vi "数据查询_仪器数据.vi"() -> ()   [LabVIEW 2016]
uses:
  <vilib>/Utility/miscctls.llb/LVRowAndColumnUnsignedTypeDef.ctl
  <vilib>/Utility/miscctls.llb/LVPointTypeDef.ctl
  SQL/database.lvlib
panel:
  in  "查询":bool
  in  "结束日期":string="2020/01/01"
  in  "起始日期":string="2010/01/01"
  in  "组合框":string(combo)
  out "数据表":string[][](table)
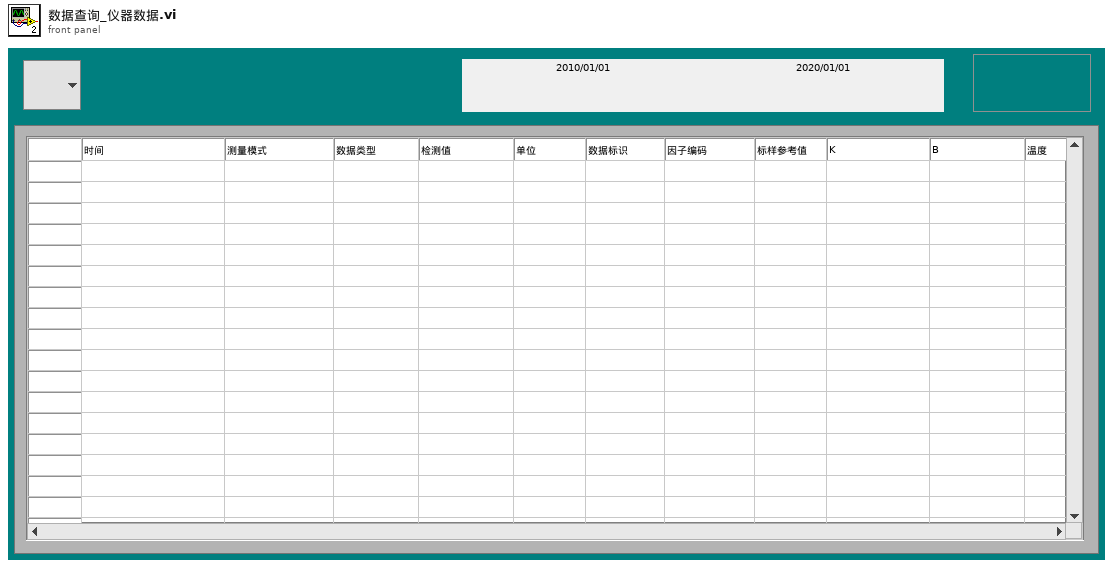
[diagram p1: front panel]
types:
  T1 = typedef "LVRowAndColumnUnsignedTypeDef.ctl" = cluster{"Row":u32, "Column":u32}
  T2 = typedef "LVPointTypeDef.ctl" = cluster{"Horizontal":i16, "Vertical":i16}
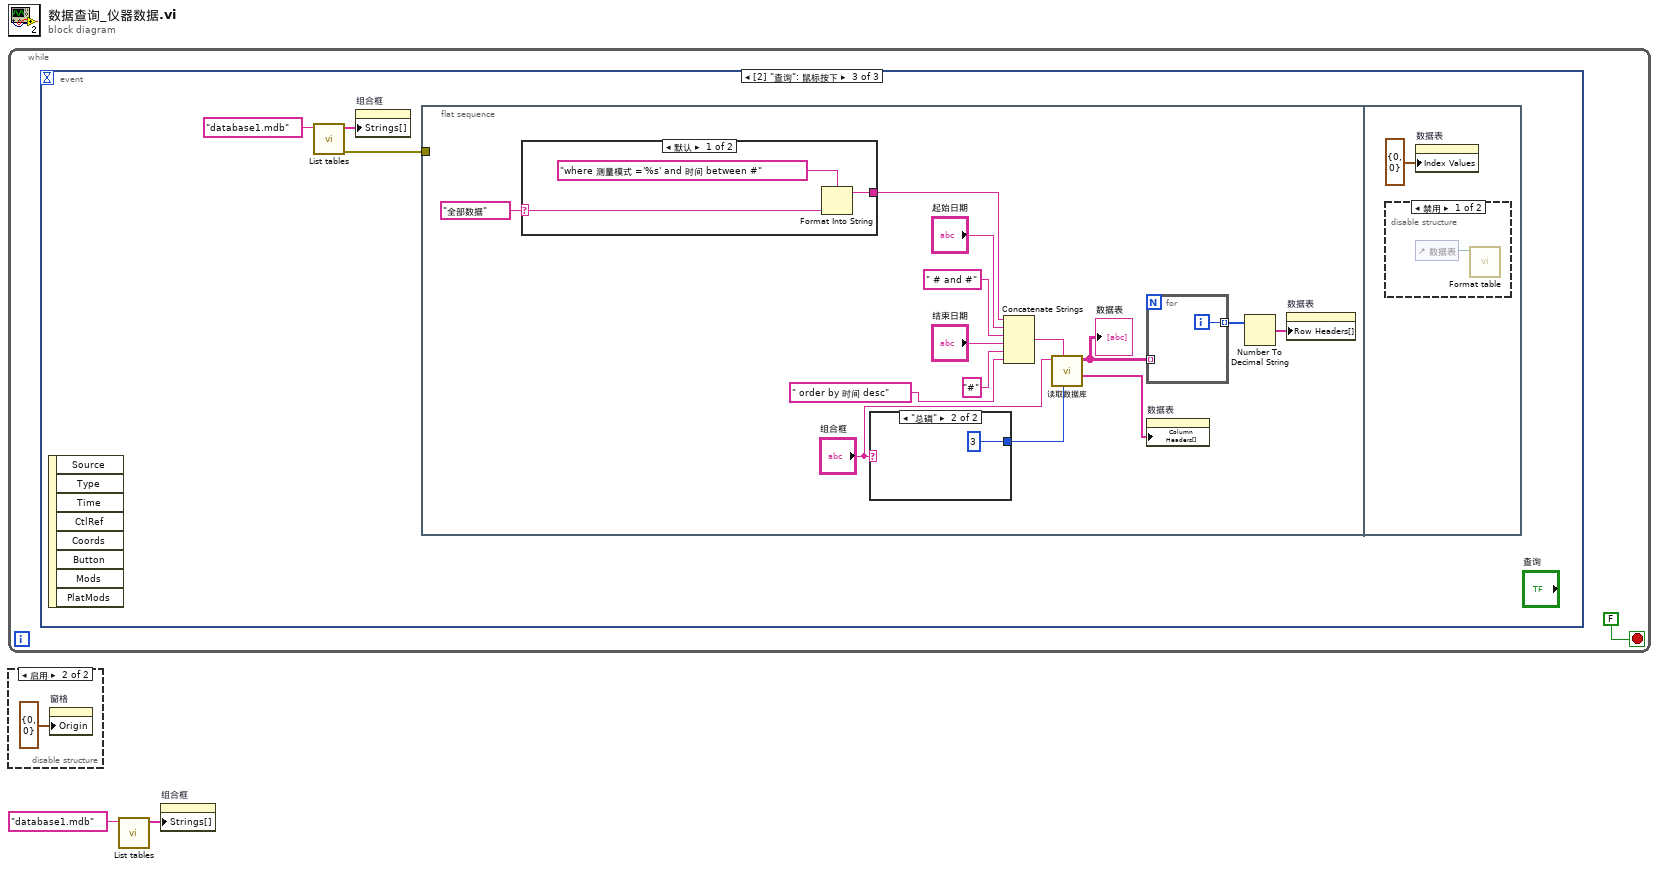
[diagram p0: block diagram]
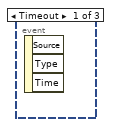
[diagram p2: hidden frame]
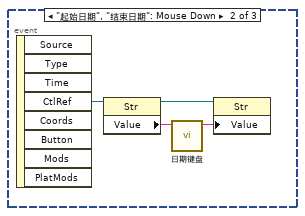
[diagram p3: hidden frame]
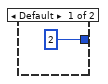
[diagram p4: hidden frame]
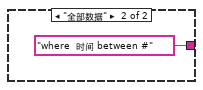
[diagram p5: hidden frame]
diagram:
  n1 = while {
    stop <- FALSE stop-if-true
    n2 = event shown="[2] \"查询\": 鼠标按下" {
      selector: _ -> [_ _ _]
      dyn-events: _ -> [_ _ _]
      timeout: _ -> [_ _ _]
      event Timeout {
        n3 = event-data() -> ()  [unwired: 1 in, 3 out]
      }
      event "起始日期", "结束日期": Mouse Down {
        n4 = event-data() -> ("CtlRef"=w7:refnum<vi>)  [unwired: 1 in, 7 out]
        n5 = property class="Str"(reference=w7) -> (reference out=w5:refnum<vi>, "Value"=w6:string)  [unwired: 1 in, 1 out]
        n6 = call "日期键盘.vi"("原值"=w6) -> ("x+y"=w4:string)  [unwired: 10 in]
        n7 = property class="Str"(reference=w5, "Value"=w4) -> ()  [unwired: 1 in, 2 out]
      }
      event "查询": Mouse Down {
        n8 = event-data() -> ()  [unwired: 1 in, 8 out]
        n9 = call "List tables.vi"("database"="database1.mdb") -> ("error out"=w8:errorcluster, "tables"=w10:string[])  [unwired: 9 in]
        n10 = property on="组合框" class="CmbBox"("Strings[]"=w10) -> ()  [unwired: 2 in, 2 out]
        n11 = flat-sequence {
          tunnel: w8 -> [_]
          frame #0 {
            n12 = case shown="默认" "全部数据" ("工作模式") {
              selector: "全部数据" ("工作模式") -> [w29 _]
              tunnel: [w27 "where  时间 between #" ("condition")] -> w13
              frame Default {
                n13 = Format Into String(format string="where 测量模式 ='%s' and 时间 between #" ("condition"), w29) -> (resulting string=w27:string)  [unwired: 2 in, 1 out]
              }
              frame "全部数据" {
              }
            }
            n14 = case shown="\"总磷\"" "组合框" {
              tunnel: [i16 2 ("精度(6)") i16 3 ("精度(6)")] -> w11
              frame Default {
              }
              frame "总磷" {
              }
            }
            n15 = Concatenate Strings(w13, "起始日期", " # and #" ("condition"), "结束日期", "#" ("condition"), " order by 时间 desc" ("字符串")) -> (w23:string)
            n16 = call "读取数据库.vi"("精度(6)"=w11, "condition"=w23, "组合框"="组合框") -> ("columns"=w19:string[], "表格"=w17:string[][])  [unwired: 5 in, 2 out]
            "数据表" <- w17
            n17 = for {
              tunnel: w17 -> [_] mode=indexing
              tunnel: [w31] -> w16 mode=indexing
              i -> [w31]
            }
            n18 = property on="数据表" class="Tbl (严格)"("Column Headers[]"=w19) -> ()  [unwired: 2 in, 2 out]
            n19 = Number To Decimal String(number=w16) -> (decimal integer string=w15:string[])  [unwired: 1 in]
            n20 = property on="数据表" class="Tbl (严格)"("Row Headers[]"=w15) -> ()  [unwired: 2 in, 2 out]
          }
          frame #1 {
            n21 = disable-structure shown="禁用" {
              frame Disabled {
                n22 = control-ref of="数据表"() -> (w33:refnum<vi>)
                n23 = call "Format table.vi"("Table输入"=w33) -> ()  [unwired: 11 in]
              }
              frame Enabled {
              }
            }
            n24 = property on="数据表" class="Tbl (严格)"("Index Values"=T1 {"Row"=0, "Column"=0} ("索引值")) -> ()  [unwired: 2 in, 2 out]
          }
        }
      }
    }
  }
  n25 = disable-structure shown="启用" {
    frame Disabled {
    }
    frame Enabled {
      n26 = property on="窗格" class="Pane"("Origin"=T2 {"Horizontal"=0, "Vertical"=0} ("原点")) -> ()  [unwired: 2 in, 2 out]
    }
  }
  n27 = call "List tables.vi"("database"="database1.mdb") -> ("tables"=w1:string[])  [unwired: 9 in, 1 out]
  n28 = property on="组合框" class="CmbBox"("Strings[]"=w1) -> ()  [unwired: 2 in, 2 out]
